vi "myRIO v1.0 Create Configuration List.vi"() -> (3 "Bitmask Array":bool[][](array[boolean]))   [LabVIEW 2021]
panel:
  # "This VI is provided for convenience so that the creation of the bitmask array used for configuring the functions is done in a single place. Therefore, any changes can be made here instead of in every single Build MUX Configuration XXX VI."
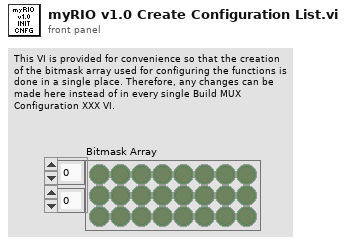
[diagram p1: front panel]
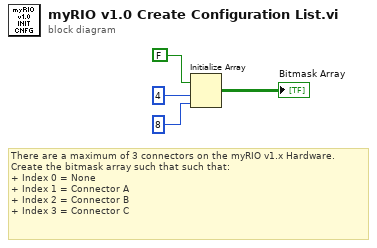
[diagram p0: block diagram]
diagram:
  # "There are a maximum of 3 connectors on the myRIO v1.x Hardware.\nCreate the bitmask array such that such that:\n+ Index 0 = None\n+ Index 1 = Connector A\n+ Index 2 = Connector B \n+ Index 3 = Connector C"
  n1 = Initialize Array(FALSE, 4 ("dimension size"), 8 ("dimension size")) -> (→"Bitmask Array":bool[][])
